vi "Lab07_subVI.vi"(3 "i":i32, 4 "duration(s)":dbl, 5 "path":path) -> (0 "end of signal":bool, 1 "sample rate (S/s)":dbl, 2 "Waveform Segment":waveform(dbl)(graph))   [LabVIEW 2025]
uses:
  <vilib>/sound2/lvsound2.llb/Sound File Info (path).vi
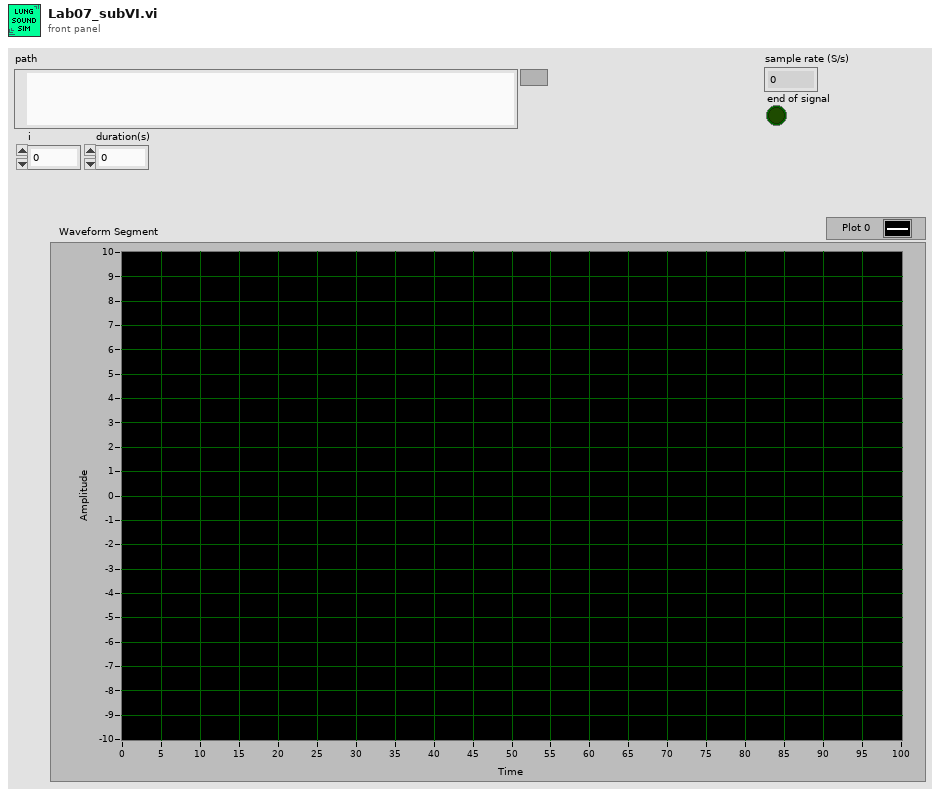
[diagram p1: front panel]
types:
  T1 = typedef "Sound Data Format.ctl" = cluster{"sample rate (S/s)":dbl, "number of channels":i32, "bits per sample":i32}
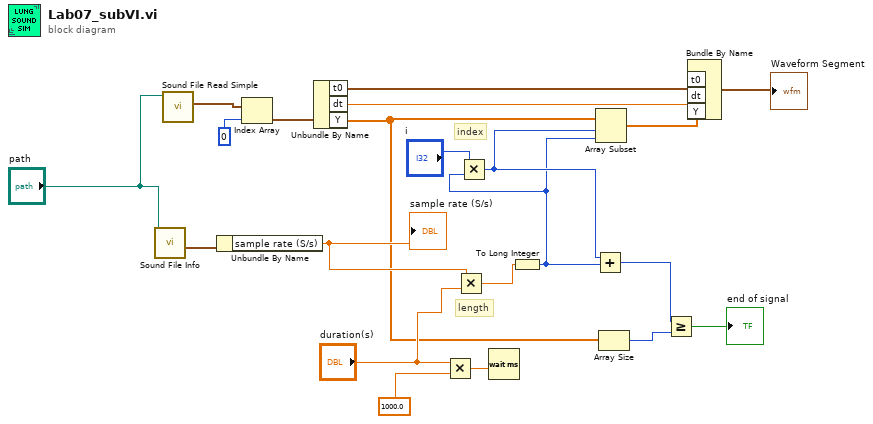
[diagram p0: block diagram]
diagram:
  # "index"
  # "length"
  n1 = call-poly <vilib>:"Sound File Info.vi"("path"="path") -> ("sound format"=w20:T1)  [unwired: 7 in, 3 out]
  n2 = call <vilib>:"Sound File Read Simple.vi"("path"="path") -> ("data"=w19:waveform(dbl)[])  [unwired: 7 in, 3 out]
  n3 = Unbundle By Name(w20) -> ("sample rate (S/s)"=w15:dbl)
  "sample rate (S/s)" <- w15
  n4 = Index Array(array=w19, index=0) -> (element=w18:waveform(dbl))
  n5 = Unbundle By Name(w18) -> ("t0"=w9:timestamp, "dt"=w8:dbl, "Y"=w4:dbl[])
  n6 = Multiply(x="duration(s)", y=1000.0) -> (x*y=w13:dbl)
  n7 = Multiply(x=w15, y="duration(s)") -> (x*y=w14:dbl)
  n8 = Wait (ms)(milliseconds to wait=w13) -> ()  [unwired: 1 out]
  n9 = To Long Integer(number=w14) -> (32bit integer=w1:i32)
  n10 = Multiply(x="i", y=w1) -> (x*y=w2:i32)
  n11 = Add(x=w2, y=w1) -> (x+y=w3:i32)
  n12 = Array Subset(array=w4, index=w2, length=w1) -> (w10:dbl[])
  n13 = Array Size(array=w4) -> (size(s)=w5:i32)
  n14 = Greater Or Equal?(x=w3, y=w5) -> (x >= y?=→"end of signal":bool)
  n15 = Bundle By Name("t0"=w9, "dt"=w8, "Y"=w10) -> (→"Waveform Segment":waveform(dbl))  [unwired: 1 in]
